vi "ButtonWait.vi"(3 "error in (no error)":errorcluster, 5 "VISA resource name":refnum<visa-resource-name>) -> (0 "error out":errorcluster, 2 "VISA resource name out":refnum<visa-resource-name>)   [LabVIEW 2009]
doc: "Waits until the user presses the button on the given cyberglove.\n\nProgram queries the cyberglove with the '?W' command until the cyberglove reports that the button has been pressed."
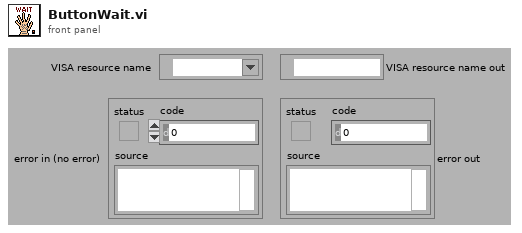
[diagram p1: front panel]
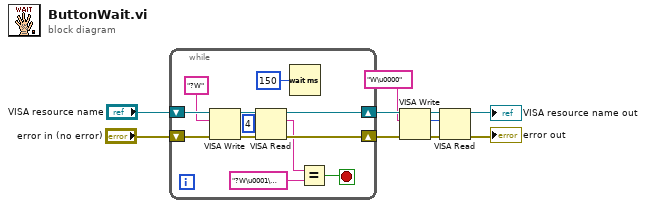
[diagram p0: block diagram]
diagram:
  n1 = while {
    shift-right: [w15] -> w8
    shift-left: "VISA resource name" -> [w21]
    shift-right: [w14] -> w7
    shift-left: "error in (no error)" -> [w20]
    stop <- w11 stop-if-true
    n2 = VISA Write(VISA resource name=w21, write buffer="?W", error in (no error)=w20) -> (VISA resource name out=w18:refnum<visa-resource-name>, error out=w17:errorcluster)  [unwired: 1 out]
    n3 = VISA Read(VISA resource name=w18, byte count=u32 4, error in (no error)=w17) -> (VISA resource name out=w15:refnum<visa-resource-name>, read buffer=w13:string, error out=w14:errorcluster)  [unwired: 1 out]
    n4 = Wait (ms)(milliseconds to wait=u32 150) -> ()  [unwired: 1 out]
    n5 = Equal?(x=w13, y="?W\u0001\u0000") -> (x = y?=w11:bool)
  }
  n6 = VISA Write(VISA resource name=w8, write buffer="W\u0000", error in (no error)=w7) -> (VISA resource name out=w5:refnum<visa-resource-name>, return count=w4:u32, error out=w3:errorcluster)
  n7 = VISA Read(VISA resource name=w5, byte count=w4, error in (no error)=w3) -> (VISA resource name out=→"VISA resource name out":refnum<visa-resource-name>, error out=→"error out":errorcluster)  [unwired: 2 out]
